vi "Drop Brick one page.vi"(7 "Map in":map{i32, T1[]}(c390), 9 "ID":i32, 11 "Array in":i32[][][](array[numeric])) -> (3 "Array out":i32[][][](array[numeric]), 5 "Map out":map{i32, T1[]}(c390))   [LabVIEW 2023]
uses:
  Cluster_Node.ctl
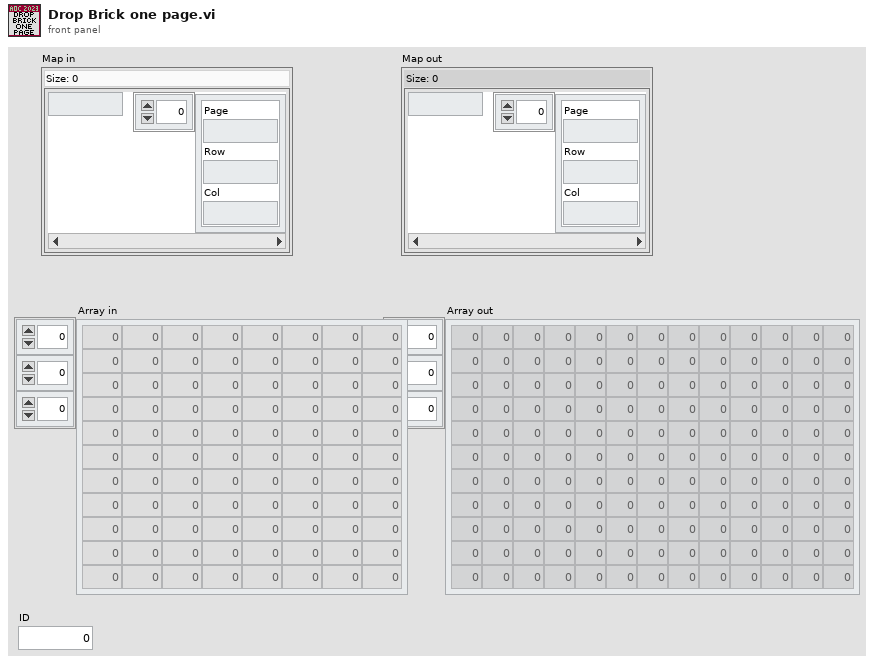
[diagram p1: front panel]
types:
  T1 = typedef "Cluster_Node.ctl" = cluster{"Page":i32, "Row":i32, "Col":i32}
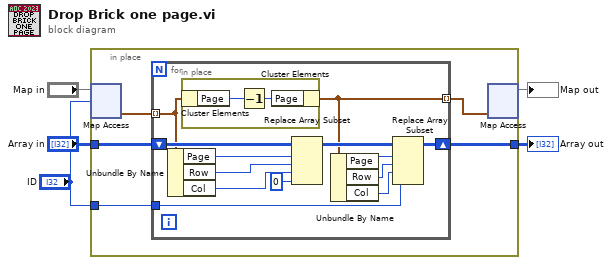
[diagram p0: block diagram]
diagram:
  n1 = in-place {
    in-place-border: "Array in" -> [w9]
    in-place-border: [w8] -> w4
    in-place-border: "ID" -> [w7]
    n2 = in-place-map #1("Map in", "ID") -> (w10:T1[])  [unwired: 1 in, 1 out]
    n3 = for {
      tunnel: w10 -> [w15] mode=indexing
      shift-right: [w18] -> w8
      shift-left: w9 -> [w23]
      tunnel: w7 -> [w16]
      tunnel: [w14] -> w6 mode=indexing
      n4 = Unbundle By Name(w15) -> ("Page"=w22:i32, "Row"=w21:i32, "Col"=w20:i32)
      n5 = in-place {
        n6 = in-place-cluster #2(w15) -> ("Page"=w25:i32)
        n7 = Decrement(x=w25) -> (x-1=w24:i32)
        n8 = in-place-cluster #2("Page"=w24) -> (w14:T1)
      }
      n9 = Replace Array Subset(array=w23, new element=0 ("new element/subarray"), index (dim 0)=w22, index (dim 1)=w21, index (dim 2)=w20) -> (w17:i32[][][])
      n10 = Unbundle By Name(w14) -> ("Page"=w13:i32, "Row"=w12:i32, "Col"=w11:i32)
      n11 = Replace Array Subset(array=w17, new element=w16, index (dim 0)=w13, index (dim 1)=w12, index (dim 2)=w11) -> (w18:i32[][][])
    }
    n12 = in-place-map #1(w6) -> (→"Map out":map{i32, T1[]})  [unwired: 1 in, 2 out]
  }
  "Array out" <- w4
